vi "AC20150928_1803_Sub_Messung#3.vi"(2 "Reset":bool, 3 "Übernehmen":bool, 4 "U_mess_in":dbl) -> (1 "Mess_Array_Out[6]":dbl[](array[numeric]))   [LabVIEW 2018]
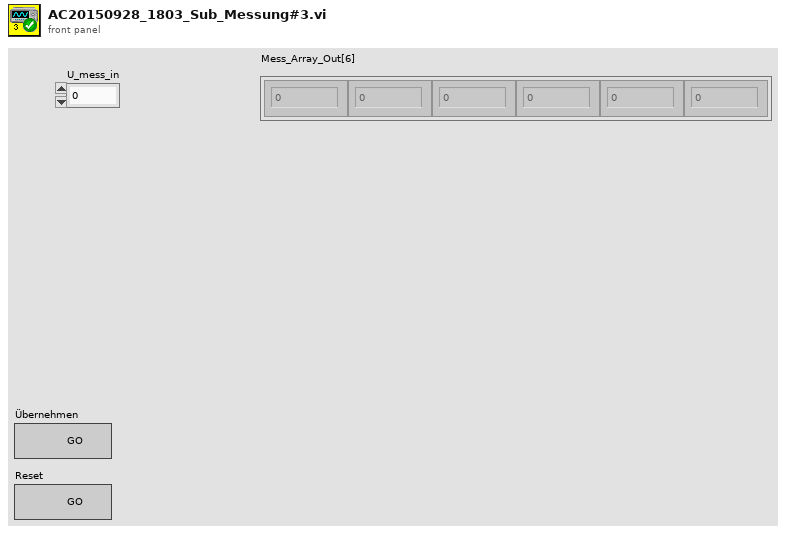
[diagram p1: front panel]
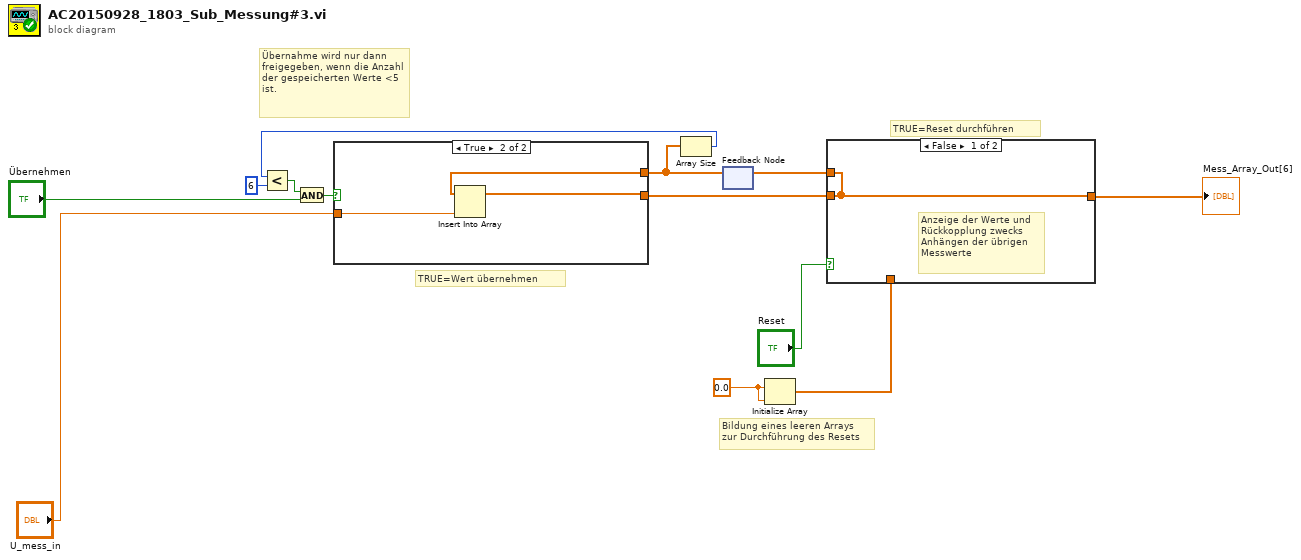
[diagram p0: block diagram]
diagram:
  w3 = 0.0
  # "Übernahme wird nur dann freigegeben, wenn die Anzahl der gespeicherten Werte <5 ist."
  # "TRUE=Wert übernehmen"
  # "TRUE=Reset durchführen"
  # "Bildung eines leeren Arrays\nzur Durchführung des Resets"
  n1 = feedback #1() -> (w8:dbl[])  [unwired: 1 in]
  n2 = Array Size(array=w8) -> (size(s)=w12:i32)
  n3 = Less?(x=w12, y=6) -> (x < y?=w11:bool)
  n4 = And(x=w11, y="Übernehmen") -> (x .and. y?=w10:bool)
  n5 = case shown="True" w10 {
    tunnel: "U_mess_in" -> [_ w17]
    tunnel: [w14 w16] -> w6
    tunnel: w8 -> [w14 w15]
    frame False {
    }
    frame True {
      n6 = Insert Into Array(array=w15, new element=w17) -> (w16:dbl[])  [unwired: 1 in]
    }
  }
  n7 = Initialize Array(w3, w3) -> (w4:dbl[])
  n8 = case shown="False" "Reset" {
    tunnel: [w18 w19] -> w5
    tunnel: w6 -> [w18 _]
    tunnel: w4 -> [_ w19]
    tunnel: [w18 w19] -> w7
    frame False {
      # "Anzeige der Werte und\nRückkopplung zwecks \nAnhängen der übrigen \nMesswerte"
    }
    frame True {
      # "Übernahme und Rückkoppeln\neines leeren Arrays zwecks Reset"
    }
  }
  "Mess_Array_Out[6]" <- w5
  n9 = feedback-in #1(w7) -> ()
